vi "零点跨度数据组合 (子VI).vi"(8 "span value":string="0", 9 "standard value":string, 10 "check value":string, 11 "污染物编码":string) -> (3 "组合输出":string)   [LabVIEW 2016, in "数据传输系统.lvlib"]
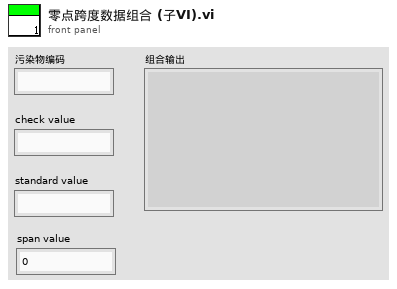
[diagram p1: front panel]
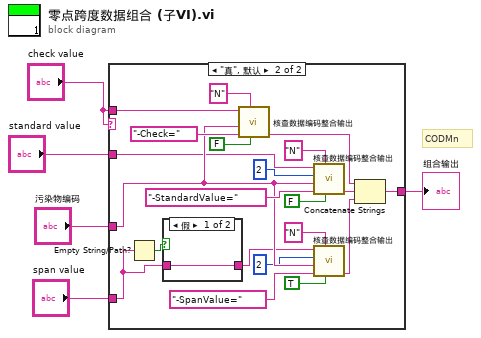
[diagram p0: block diagram]
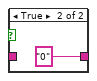
[diagram p3: hidden frame]
diagram:
  # "CODMn"
  n1 = case shown="\"真\", 默认" "check value" {
    tunnel: "check value" -> [w6 w26]
    tunnel: [w6 w23] -> w2
    tunnel: "standard value" -> [_ w10]
    tunnel: "污染物编码" -> [_ w13]
    tunnel: "span value" -> [_ w7]
    frame "" {
    }
    frame "真", Default {
      n2 = Empty String/Path?(string/path=w7) -> (empty?=w9:bool)
      n3 = case shown="假" w9 {
        tunnel: [w28 "0"] -> w8
        tunnel: w7 -> [w28 _]
        frame False {
        }
        frame True {
        }
      }
      n4 = call "核查数据编码整合输出.vi"("字段结束"=FALSE, "数据标识"="N" ("字符串"), "数据类型"="-Check=", "污染物编码"=w13, "数据值"=w26) -> ("编码输出"=w24:string)  [unwired: 6 in]
      n5 = call "核查数据编码整合输出.vi"("字段结束"=FALSE, "数据标识"="N" ("字符串"), "数据类型"="-StandardValue=", "污染物编码"=w13, "数据精度"=2, "数据值"=w10) -> ("编码输出"=w20:string)  [unwired: 5 in]
      n6 = call "核查数据编码整合输出.vi"("字段结束"=TRUE, "数据标识"="N" ("字符串"), "数据类型"="-SpanValue=", "污染物编码"=w13, "数据精度"=2, "数据值"=w8) -> ("编码输出"=w17:string)  [unwired: 5 in]
      n7 = Concatenate Strings(w24, w20, w17) -> (w23:string)
    }
  }
  "组合输出" <- w2
